vi "setVertical.vi"(7 "Chn":string, 8 "error in (no error)":errorcluster, 9 "Dc Offset":dbl, 10 "Range [V]":dbl, 11 "ScopeKeysight in":refnum<class "ScopeKeysight.lvclass">) -> (0 "error out":errorcluster, 3 "ScopeKeysight out":refnum<class "ScopeKeysight.lvclass">)   [LabVIEW 2023, in "ScopeKeysight.lvclass"]
doc: "<b>Author:</b> Wolfgang\n<b>Description:</b> configure the vertical range of a channel"
uses:
  ScopeKeysight.lvclass
  ScopeKeysight.lvclass/ScopeKeysight.ctl
  Driver/Keysight-DSQx3014T.lvlib
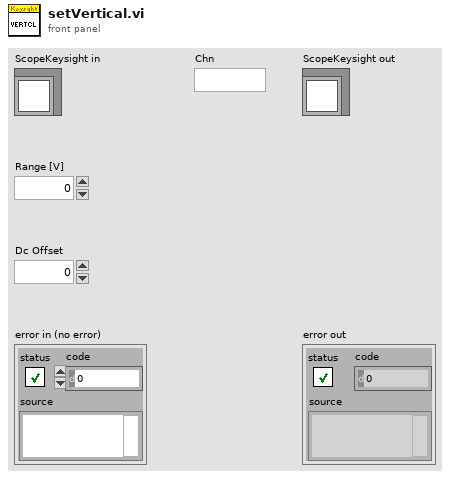
[diagram p1: front panel]
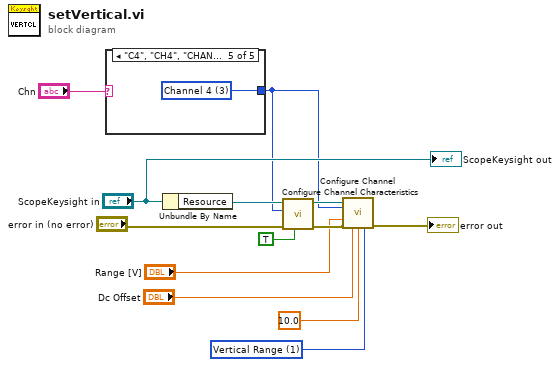
[diagram p0: block diagram]
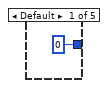
[diagram p2: hidden frame]
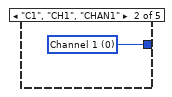
[diagram p3: hidden frame]
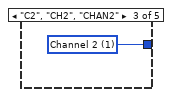
[diagram p4: hidden frame]
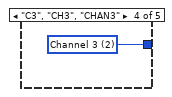
[diagram p5: hidden frame]
diagram:
  w2 = 1 items=["Vertical Scale", "Vertical Range"] ("Vertical Setting (1: Vertical Range)")
  n1 = case shown="\"C4\", \"CH4\", \"CHAN4\"" "Chn" {
    tunnel: [0 ("Channel Name (0: Channel 1)") w15 w16 w17 w18] -> w5
    frame Default {
    }
    frame "C1", "CH1", "CHAN1" {
      w15 = 0 items=["Channel 1", "Channel 2", "Channel 3", "Channel 4"] ("Channel Name (0: Channel 1)")
    }
    frame "C2", "CH2", "CHAN2" {
      w16 = 1 items=["Channel 1", "Channel 2", "Channel 3", "Channel 4"] ("Channel Name (0: Channel 1)")
    }
    frame "C3", "CH3", "CHAN3" {
      w17 = 2 items=["Channel 1", "Channel 2", "Channel 3", "Channel 4"] ("Channel Name (0: Channel 1)")
    }
    frame "C4", "CH4", "CHAN4" {
      w18 = 3 items=["Channel 1", "Channel 2", "Channel 3", "Channel 4"] ("Channel Name (0: Channel 1)")
    }
  }
  n2 = Unbundle By Name("ScopeKeysight in") -> ("Resource"=w12:refnum<visa-resource-name>)
  n3 = call "Configure Channel Characteristics.vi"("Enable Vernier (F: Disable)"=TRUE, "error in (no error)"="error in (no error)", "Channel Name (0: Channel 1)"=w5, "VISA resource name"=w12) -> ("error out"=w7:errorcluster, "VISA resource name out"=w8:refnum<visa-resource-name>)  [unwired: 6 in]
  n4 = call "Configure Channel.vi"("VISA resource name"=w8, "Channel Name (0: Channel 1)"=w5, "Vertical Range (40.0 V)"="Range [V]", "error in (no error)"=w7, "Vertical Offset (0.0)"="Dc Offset", "Probe Attenuation (1.0)"=10.0, "Vertical Setting (1: Vertical Range)"=w2) -> ("error out"=→"error out":errorcluster)  [unwired: 7 in, 1 out]
  "ScopeKeysight out" <- "ScopeKeysight in"
